vi "FlexibleBlock - Finite PCM Acquisition(Slave) - I2S.vi"() -> ()   [LabVIEW 2021]
uses:
  <vilib>/PDM Acquisition Toolkit/host/Classes/Session/Controls/Logic Levels.ctl
  <vilib>/PDM Acquisition Toolkit/shared/controls/PCM Data Format Configuration.ctl
  <vilib>/PDM Acquisition Toolkit/shared/controls/Digital Edge.ctl
  <vilib>/PDM Acquisition Toolkit/shared/controls/PCM Bit Endianness.ctl
  <vilib>/PDM Acquisition Toolkit/shared/controls/PCM Data Justification.ctl
  <vilib>/PDM Acquisition Toolkit/shared/controls/PCM Frame Sync Control.ctl
  Program Files/National Instruments/LabVIEW 2021/examples/PDM Acquisition Toolkit/subVIs/PCM Interface Type.ctl
  Users/Admin/Desktop/Release audio branch/Audio/audio_d/audio_MeasurementService/source/measurements/ac/audio_acMeasurement/Measurement Results.ctl
  <vilib>/addons/_NISVFA/_Shared subVIs/Controls/svc_Window.ctl
  <vilib>/PDM Acquisition Toolkit/host/Classes/Tasks/PDM Tasks/Controls/Acquisition Mode.ctl
  <vilib>/addons/_NISVFA/_Shared subVIs/Common/SVL Set dB Reference (N Ch - 1 Ref).vi
  <vilib>/addons/Sound and Vibration/svt_Level/SVL AC & DC Level (Time) (N Ch).vi
  <vilib>/addons/Sound and Vibration/svt_Single Tone Measurements/SVT Spurious Free Dynamic Range (Frequency) (1 Ch).vi
  <vilib>/addons/_NISVFA/_Spectrum Processing/SVFA Unit Conversion (Complex) (1 Ch).vi
  <vilib>/addons/_NISVFA/_Shared subVIs/Common/SVL Set dB Reference (1 Ch).vi
  <vilib>/addons/Sound and Vibration/svt_Level/SVL AC & DC Level (Time) (1 Ch).vi
  <vilib>/addons/_NISVFA/_Spectrum Processing/SVFA Get Spectrum Subset.vi
  <vilib>/addons/_NISVFA/_Spectrum Processing/SVFA Get Spectrum Subset (Complex) (1 Ch).vi
  <vilib>/addons/_NISVFA/_Shared subVIs/Common/svc_Window Parameters.vi
  <vilib>/addons/_NISVFA/_Shared subVIs/Common/svc_Extract Single Tone Information (complex).vi
  <vilib>/addons/_NISVFA/_Shared subVIs/Common/svc_Check Frequency Range in Spectrum.vi
  <vilib>/addons/_NISVFA/_Spectrum Processing/SVFA Spectrum Peak Search.vi
  <vilib>/addons/_NISVFA/_Spectrum Processing/SVFA Spectrum Peak Search (1 Ch).vi
  <vilib>/addons/_NISVFA/_Shared subVIs/Common/svc_Spectrum Units.vi
  <vilib>/addons/_NISVFA/_Shared subVIs/Common/svc_Log View for Spectrum (1Ch).vi
  <vilib>/addons/_NISVFA/_Spectrum Processing/SVFA Unit Conversion (1 Ch).vi
  <vilib>/addons/_NISVFA/_Shared subVIs/Common/svc_Complex Datatype Defaults.vi
  <vilib>/addons/_NISVFA/_Shared subVIs/Common/svc_Build Unit Label for Frequency Range.vi
  <vilib>/addons/_NISVFA/_Shared subVIs/Common/SVL Set dB Reference (variant).vi
  <vilib>/addons/_NISVFA/_Shared subVIs/Common/svc_Get SV Channel Info.vi
  <vilib>/Analysis/baseanly.llb/Mean.vi
  <vilib>/Analysis/baseanly.llb/Mean (DBL).vi
  <vilib>/addons/_NISVFA/_Shared subVIs/Windowing/svfa_Scaled Time Domain Window (Array).vi
  <vilib>/addons/_NISVFA/_Spectrum Processing/SVFA Get Tone Amplitude and Phase (1 Ch).vi
  <vilib>/addons/_NISVFA/_Spectrum Processing/subVIs/svfa_Compute Complex Spectrum for Export.vi
  <vilib>/addons/_NISVFA/_Shared subVIs/Common/svc_Check Frequency Range in Bandwidth.vi
  <vilib>/addons/_NISVFA/_Shared subVIs/Common/svc_Convert Start and Stop to Start Index and Length.vi
  <vilib>/addons/_NISVFA/_Spectrum Processing/subVIs/svfa_Spectrum Peak Search.vi
  <vilib>/addons/_NISVFA/_Shared subVIs/Common/svc_Format Value (DBL).vi
  <vilib>/addons/_NISVFA/_Shared subVIs/Common/svc_Get Weighting Enum and Labels.vi
  <vilib>/addons/_NISVFA/_Shared subVIs/Common/svc_Engineering Units to Unit Label.vi
  <vilib>/addons/_NISVFA/_Shared subVIs/Common/svc_Surround NonAlpha String with Parentheses.vi
  <vilib>/dlg_ctls.llb/Space Constant.vi
  <vilib>/addons/_NISVFA/_Shared subVIs/Common/svc_Unwrap Phase.vi
  <vilib>/addons/_NISVFA/_Shared subVIs/Common/svc_Convert Spectrum Array to dB.vi
  <vilib>/addons/_NISVFA/_Spectrum Processing/subVIs/svfa_Conversion Utility (spectrum info).vi
  <vilib>/addons/_NISVFA/_Shared subVIs/Common/svc_Unit Label to Engineering Units.vi
  <vilib>/addons/_NISVFA/_Spectrum Processing/subVIs/svfa_Spectrum Info Window to windowTd Type Def.vi
  <vilib>/Analysis/4window.llb/Force Window.vi
  <vilib>/Analysis/4window.llb/Force Window (DBL).vi
  <vilib>/Analysis/4window.llb/Exponential Window.vi
  <vilib>/Analysis/4window.llb/Exponential Window (DBL).vi
  <vilib>/addons/_NISVFA/_Spectrum Processing/subVIs/svfa_Window Frequency Response.vi
  <vilib>/addons/_NISVFA/_Spectrum Processing/subVIs/svfa_Window Frequency Response (double array).vi
  <vilib>/Analysis/baseanly.llb/Dot Product.vi
  <vilib>/Analysis/baseanly.llb/Complex Dot Product.vi
  <vilib>/addons/_NISVFA/_Spectrum Processing/subVIs/svfa_Peak Rough Search Indices.vi
  <vilib>/addons/_NISVFA/_Shared subVIs/Common/svc_Unit Label Lexical Class.vi
  <vilib>/addons/_NISVFA/_Spectrum Processing/subVIs/svfa_Peak to RMS to Peak2Peak.vi
  <vilib>/addons/_NISVFA/_Spectrum Processing/subVIs/svfa_Mag to Mag2.vi
  <vilib>/addons/_NISVFA/_Spectrum Processing/subVIs/svfa_Linear to dB.vi
  <vilib>/addons/_NISVFA/_Spectrum Processing/subVIs/svfa_dBrefA to dBrefB.vi
  <vilib>/addons/_NISVFA/_Spectrum Processing/subVIs/svfa_Spectrum to Spectral Density.vi
  <vilib>/addons/_NISVFA/_Spectrum Processing/subVIs/svfa_Rect Window Frequency Response.vi
  <vilib>/addons/_NISVFA/_Spectrum Processing/subVIs/svfa_Cosine Window Coefficients.vi
  <vilib>/PDM Acquisition Toolkit/host/API/Public/Create Tasks/Create PCM Input Task.vi
  <vilib>/PDM Acquisition Toolkit/host/API/Public/Configure/Timing/Configure Timing - PCM Input Slave.vi
  <vilib>/PDM Acquisition Toolkit/host/API/Public/Configure/PDM Channel/Configure Microphone Sensitivity FSPA - PCM Input Task.vi
  <vilib>/PDM Acquisition Toolkit/host/API/Public/Utility/Configure Simulation Mode - PCM Input Task.vi
  <vilib>/PDM Acquisition Toolkit/host/API/Public/Start/Start PCM Input Task.vi
  <vilib>/PDM Acquisition Toolkit/host/API/Public/Read/Read PCM Input Waveform.vi
  <vilib>/measure/matone.llb/Extract Single Tone Information N Chan.vi
  <vilib>/PDM Acquisition Toolkit/host/API/Public/Clear/Clear PCM Input Task.vi
  <vilib>/addons/Sound and Vibration/svt_Weighting/SVT Weighting Filter (N Ch).vi
  <vilib>/addons/_NISVFA/_Shared subVIs/Common/svc_Caller VI Returned in Error Source.vi
  <vilib>/addons/_NISVFA/_Shared subVIs/Common/svc_Get Window Info.vi
  <vilib>/Analysis/0measdsp.llb/Scaled Time Domain Window.vi
  <vilib>/Analysis/0measdsp.llb/Scaled Time Domain Window (DBL).vi
  <vilib>/Utility/error.llb/Error Cluster From Error Code.vi
  <vilib>/Analysis/baseanly.llb/Std Deviation and Variance.vi
  <vilib>/addons/Sound and Vibration/svt_Single Tone Measurements/SVT Gain (Time) (1 Ch).vi
  <vilib>/addons/Sound and Vibration/svt_Distortion/SVT SNR without Harmonics (Frequency) (1 Ch).vi
  <vilib>/addons/Sound and Vibration/svt_Single Tone Measurements/SVT Dynamic Range (Frequency) (1 Ch).vi
  <vilib>/addons/Sound and Vibration/svt_Distortion/subVIs/sv_Check Data Valid (Audio) (1 Ch).vi
  <vilib>/addons/_NISVFA/_Shared subVIs/Common/svc_Convert Frequency to Frequency String.vi
  <vilib>/Analysis/4window.llb/window parameters.vi
  <vilib>/Analysis/4window.llb/Window Properties.vi
  <vilib>/Analysis/4window.llb/Window Properties by Name.vi
  <vilib>/addons/_NISVFA/_Spectrum Processing/subVIs/svfa_Spectrum Peak Tone Search and Estimation (complex).vi
  <vilib>/measure/masignal.llb/Tones and Noise Waveform.vi
  <vilib>/addons/_NISVFA/_Shared subVIs/Common/svc_FFT with Window.vi
  <vilib>/Analysis/1siggen.llb/Square Wave.vi
  <vilib>/addons/_NISVFA/_Spectrum Processing/subVIs/svfa_Three Finger Peak Search.vi
  <vilib>/addons/Sound and Vibration/svt_Distortion/subVIs/sv_Peak View Amplitude (1 Ch).vi
  <vilib>/PDM Acquisition Toolkit/host/API/PDM Acquisition Toolkit.lvlib
  <vilib>/PDM Acquisition Toolkit/host/Classes/Tasks/PDM Tasks/PDM Task.lvclass
  <vilib>/measure/NI_MAPro.lvlib
  <vilib>/addons/Sound and Vibration/svt_Single Tone Measurements/SoundVib_SingleTone.lvlib
  <vilib>/addons/Sound and Vibration/svt_Distortion/SoundVib_Distortion.lvlib
  <vilib>/addons/Sound and Vibration/svt_Weighting/SoundVib_ABCWeighting.lvlib
  <vilib>/PDM Acquisition Toolkit/host/Classes/Session/DecoderSession.lvclass
  <vilib>/PDM Acquisition Toolkit/shared/PDM Shared.lvlib
  Users/Admin/Desktop/Release audio branch/Audio/audio_d/audio_MeasurementService/source/measurements/ac/audio_acMeasurement/audio_acMeasurement.lvlib
panel:
  out "FreqDomainGraph":cluster{"x0":dbl, "dx":dbl, "magnitude":dbl[]}(graph) caption="AC"
  out "output cluster":T1
  out "error out":errorcluster
  in  "Latch Delay(ns)":sgl
  in  "PCM Interfaces":T2
  out "elements remaining":u32[](array[numeric])=[26]
  out "Frame Sync Clock Control":T3={"Frame Length"=64, "Frame Sync Pulse Width"=32, "Bit Clock Edge  Sync"=enum."Falling"}
  out "PCM Data Configuration":T5={"Frame Sync Edge for Channel 0"=enum."Falling", "Channel Count Per Frame"=2, "Channel Length"=32, "Bit Depth"=24, "Channel 0 Offset"=1, "Endianness"=enum."MSB First", "Data Justification"=enum."Left Justified"}
  in  "Bit clock rate":u32=12288000 format="%.4p"
  in  "logic level":T8
  out "Requested Sampling Rate":dbl=192000.0 format="%#_6p"
  out "detected phases (deg)":dbl[](array[numeric])=[48.77177137902379, 163.50683535190996] format="%.2p"
  out "detected amplitudes":dbl[](array[numeric])=[0.002127835538874218, 39.382575869286214] format="%.2p"
  out "detected frequencies":dbl[](array[numeric])=[87725.90443160792, 99.99819936214169] format="%.2p"
  in  "simulation mode":bool
  out "PCM Data":waveform(dbl)[](graph)=[{"t0"=timestamp(0 s since 1904-01-01), "dt"=5.208333277550992e-06, "Y"=array[4000 elements], "attributes"=variant("NI_ChannelName"=variant(string "PCMI0.0"))}, {"t0"=timestamp(0 s since 1904-01-01), "dt"=5.208333277550992e-06, "Y"=array[4000 elements], "attributes"=variant("NI_ChannelName"=variant(string "PCMI0.1"))}]
  in  "microphone sensitivity (dB/Pa)":dbl=0.34762
  in  "number of words":i32=19200
  in  "channel list":string="7820\\PCMi 0"
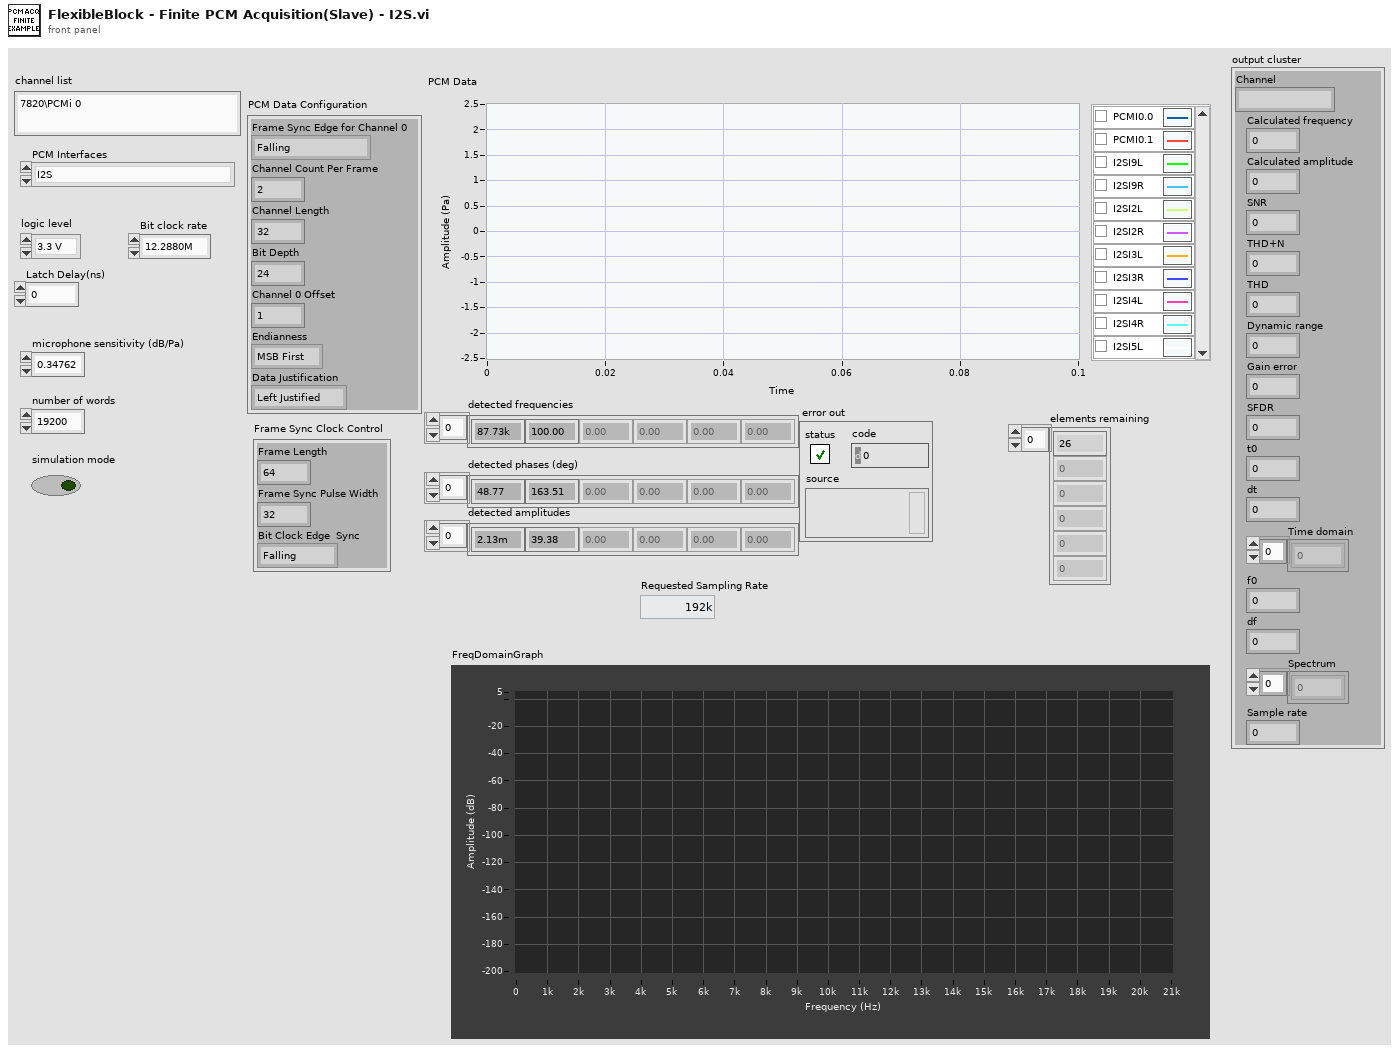
[diagram p1: front panel]
types:
  T1 = typedef "audio_acMeasurement.lvlib/Measurement Results.ctl" = cluster{"Channel":string, "Calculated frequency":dbl, "Calculated amplitude":dbl, "SNR":dbl, "THD+N":dbl, "THD":dbl, "Dynamic range":dbl, "Gain error":dbl, "SFDR":dbl, "t0":dbl, "dt":dbl, "Time domain":dbl[], "f0":dbl, "df":dbl, "Spectrum":dbl[], "Sample rate":u32}
  T2 = typedef "PCM Interface Type.ctl" = enum16{"I2S", "Left Justified", "Right Justified", "TDM 4 Channel", "TDM 6 Channel", "TDM 8 Channel", "DSP mode", "DSP mode with 1 bit delay", "PCM Short Frame", "PCM Long Frame"}
  T3 = typedef "PDM Shared.lvlib/PCM Frame Sync Control.ctl" = cluster{"Frame Length":u16, "Frame Sync Pulse Width":u16, "Bit Clock Edge  Sync":T4}
  T4 = typedef "PDM Shared.lvlib/Digital Edge.ctl" = enum8{"Rising", "Falling"}
  T5 = typedef "PDM Shared.lvlib/PCM Data Format Configuration.ctl" = cluster{"Frame Sync Edge for Channel 0":T4, "Channel Count Per Frame":u8, "Channel Length":u16, "Bit Depth":u8, "Channel 0 Offset":u16, "Endianness":T6, "Data Justification":T7}
  T6 = typedef "PDM Shared.lvlib/PCM Bit Endianness.ctl" = enum16{"MSB First", "LSB First"}
  T7 = typedef "PDM Shared.lvlib/PCM Data Justification.ctl" = enum16{"Left Justified", "Right Justified"}
  T8 = typedef "PDM Acquisition Class Library.lvlib/DecoderSession.lvclass/Logic Levels.ctl" = enum16{"3.3 V", "1.8 V", "1.2 V"}
  T9 = cluster{"Channel":string, "Calculated frequency":dbl, "Calculated amplitude":dbl, "SNR":dbl, "THD+N":dbl, "THD":dbl, "Dynamic range":dbl, "Gain error":dbl, "SFDR":dbl, "t0":dbl, "dt":dbl, "Time domain":dbl[], "f0":dbl, "df":dbl, "Spectrum":dbl[], "Sample rate":u32}
  T10 = enum16{"no change", "spectrum", "spectral density"}
  T11 = cluster{"linear/dB":enum16{"no change", "linear", "dB"}, "dB reference (0: no change)":dbl, "power/magnitude":enum16{"no change", "power", "magnitude"}, "view":enum16{"no change", "rms", "peak", "peak-peak"}}
  T12 = cluster{"start frequency":dbl, "stop frequency":dbl}
  T13 = cluster{"gain units":enum16{"dB", "linear ratio"}, "detected fundamental amplitude units":enum16{"EU rms", "EU peak", "EU peak-peak"}}
  T14 = typedef "svc_Window.ctl" = u32
  T15 = cluster{"SNR units":enum16{"dB", "linear ratio", "%"}, "detected fundamental amplitude units":enum16{"EU rms", "EU peak", "EU peak-peak"}}
  T16 = typedef "PDM Acquisition Class Library.lvlib/PDM Task.lvclass/Acquisition Mode.ctl" = enum16{"Finite", "Continuous"}
  T17 = typedef "PDM Acquisition Class Library.lvlib/PCM Input Task.lvclass/DVR PCM Input Task.ctl" = refnum<data-value>
  T18 = typedef "svc_Spectrum Info.ctl" = cluster{"channel name":string, "description":string, "x-axis units":T19, "spectral info":cluster{"spectrum type":T20, "linear/dB":enum16{"linear", "dB"}, "window":u16, "window size":i32, "FFT size":i32}, "engineering units":T21, "custom label":string, "dB reference [EU]":dbl, "peak units":enum16{"rms", "peak", "peak-peak"}, "weighting filter":T22, "spectral density?":bool, "unit label":string, "spectrum skewed?":bool, "complimentary spectrum units":T23}
  T19 = typedef "svc_X-Axis Units.ctl" = u16
  T20 = typedef "svc_Spectrum Type.ctl" = enum16{"FFT Spectrum [complex]", "Amplitude [Magnitude]", "Power [Magnitude^2]", "Cross Spectrum [complex]", "Frequency Response [Complex]"}
  T21 = typedef "svc_Engineering Units Text Ring.ctl" = u16
  T22 = typedef "svc_Weighting Filter Text Ring.ctl" = u16
  T23 = typedef "svc_Complimentary Spectrum Units.ctl" = enum16{"none", "radians", "degrees", "cycles", "imaginary"}
  T24 = cluster{"complex spectrum response":cluster{"f0":dbl, "df":dbl, "complex spectrum":cdb[]}, "spectrum info":T18}
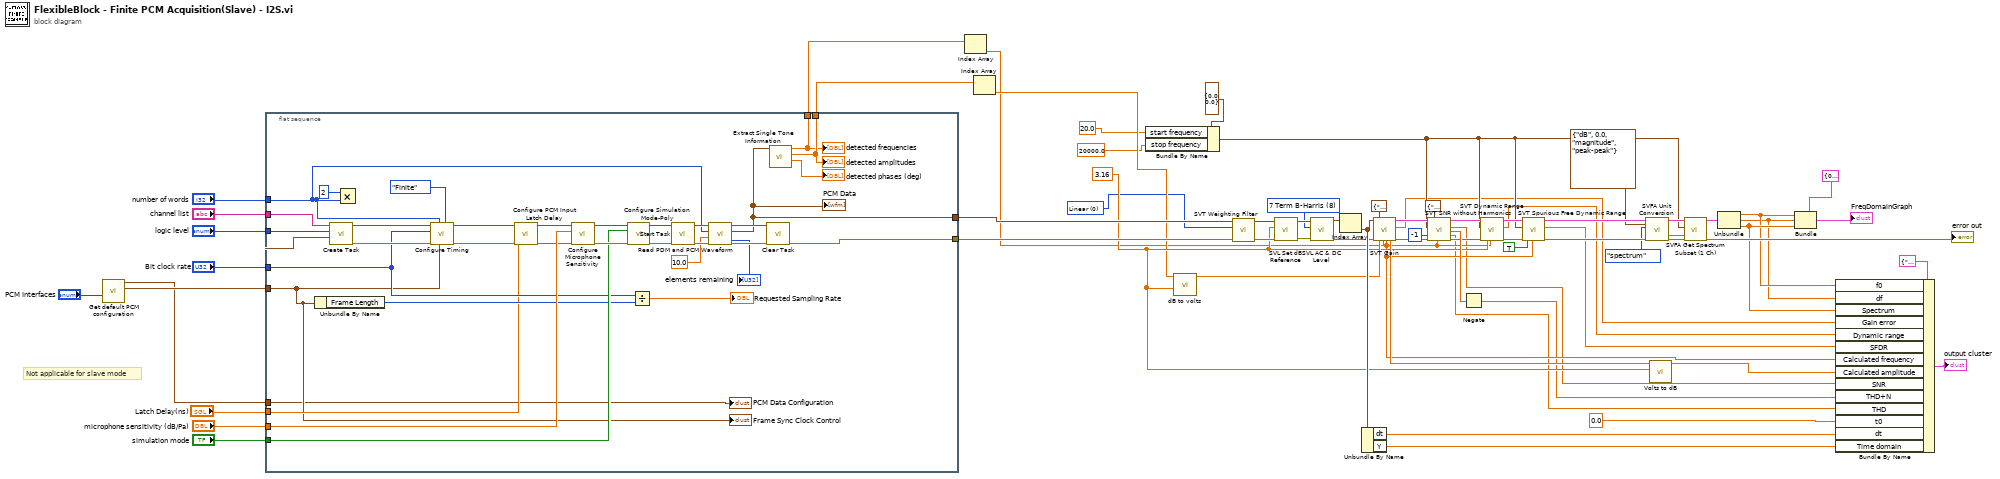
[diagram p0: block diagram]
diagram:
  w21 = u16 0 items=["Linear", "A-weighting", "B-weighting", "C-weighting"] ("weighting")
  w24 = 3.16 ("start frequency")
  w44 = T14 8 items=["None"=0, "Hanning"=1, "Hamming"=2, "Blackman-Harris"=3, "Exact Blackman"=4, "Blackman"=5, "Flat Top"=6, "4 Term B-Harris "=7, "7 Term B-Harris"=8, "Low Sidelobe"=9, "Force"=64, "Exponential"=65, "Blackman Nuttall"=11, "Triangle"=30, "Bartlett-Hanning"=31, "Bohman"=32, "Parzen"=33, "Welch"=34, "Kaiser"=60, "Dolph-Chebyshev"=61, "Gaussian"=62] ("window")
  # "Not applicable for slave mode"
  n1 = call "Get default PCM configuration.vi"("PCM Interfaces"="PCM Interfaces") -> ("Frame Sync Clock Control"=w62:T3, "PCM Data Configuration"=w61:T5)  [unwired: 9 in]
  n2 = flat-sequence {
    tunnel: "logic level" -> [w104]
    tunnel: "channel list" -> [w103]
    tunnel: "microphone sensitivity (dB/Pa)" -> [w101]
    tunnel: "simulation mode" -> [w94]
    tunnel: "Bit clock rate" -> [w85]
    tunnel: "number of words" -> [w78]
    tunnel: "Latch Delay(ns)" -> [w77]
    tunnel: w62 -> [w76]
    tunnel: w61 -> [w75]
    tunnel: [w74] -> w28
    tunnel: [w73] -> w27
    tunnel: [w72] -> w26
    tunnel: [w71] -> w25
    frame #0 {
      n3 = Unbundle By Name(w76) -> ("Frame Length"=w81:u16)
      n4 = call-poly <vilib>:"Create Task.vi"("PCM data configuration"=w75, "logic level"=w104, "channel list"=w103) -> ("error out"=w92:errorcluster, "PCM input task out"=w91:T17)  [unwired: 7 in]
      n5 = Multiply(x=2, y=w78) -> ()  [unwired: 1 out]
      n6 = call-poly <vilib>:"Configure Timing.vi"("acquisition mode"=Acquisition_Mode."Finite", "Frame Sync Clock Control"=w76, "number of words per channel"=w78, "error in"=w92, "Bit Clock rate"=w85, "PCM input task in"=w91) -> ("error out"=w90:errorcluster, "PCM input task out"=w83:T17)  [unwired: 4 in]
      n7 = call <vilib>:"Configure PCM Input Latch Delay.vi"("error in"=w90, "Latch Delay(ns)"=w77, "PCM input task in"=w83) -> ("error out"=w89:errorcluster, "PCM input task out"=w88:T17)  [unwired: 6 in, 1 out]
      n8 = call-poly <vilib>:"Configure Microphone Sensitivity.vi"("error in"=w89, "microphone sensitivity (FS/Pa)"=w101, "PCM input task in"=w88) -> ("error out"=w96:errorcluster, "PCM input task out"=w95:T17)  [unwired: 7 in]
      n9 = call-poly <vilib>:"Configure Simulation Mode-Poly.vi"("error in"=w96, "simulation mode"=w94, "PCM Input Task in"=w95) -> ("error out"=w86:errorcluster, "PCM Input Task out"=w87:T17)  [unwired: 7 in]
      n10 = Divide(x=w85, y=w81) -> (x/y=→"Requested Sampling Rate":dbl)
      n11 = call-poly <vilib>:"Start Task.vi"("error in"=w86, "PCM input task in"=w87) -> ("error out"=w100:errorcluster, "PCM input task out"=w99:T17)  [unwired: 8 in]
      n12 = call-poly <vilib>:"Read PDM and PCM Waveform.vi"("error in"=w100, "timeout"=10.0, "words per channel"=w78, "PCM input task In"=w99) -> ("error out"=w98:errorcluster, "PCM waveforms"=w73:waveform(dbl)[], "PCM input task out"=w97:T17, "elements remaining"=→"elements remaining":u32[])  [unwired: 4 in]
      "PCM Data" <- w73
      n13 = call-poly <vilib>:"Clear Task.vi"("error in"=w98, "PCM input task in"=w97) -> ("error out"=w74:errorcluster)  [unwired: 9 in]
      n14 = call-poly <vilib>:"Extract Single Tone Information.vi"("time signals in"=w73) -> ("detected phases (deg)"=→"detected phases (deg)":dbl[], "detected amplitudes"=w72:dbl[], "detected frequencies"=w71:dbl[])  [unwired: 5 in, 3 out]
      "detected frequencies" <- w71
      "detected amplitudes" <- w72
      "PCM Data Configuration" <- w75
      "Frame Sync Clock Control" <- w76
    }
  }
  n15 = Index Array(array=w25) -> (element=w22:dbl)  [unwired: 1 in]
  n16 = Index Array(array=w26) -> (element=w23:dbl)  [unwired: 1 in]
  n17 = Bundle By Name(cluster=T12 {"start frequency"=0.0, "stop frequency"=0.0} ("frequency range"), "start frequency"=20.0, "stop frequency"=20000.0 ("start frequency")) -> (w33:T12)
  n18 = call "dB to volts.vi"("Full scale range"=w24, "Voltage(dB)"=w23) -> ("Voltage(volts)"=w37:dbl)  [unwired: 9 in]
  n19 = call-poly <vilib>:"SVT Weighting Filter.vi"("error in (no error)"=w28, "weighting"=w21, "scaled signals [EU]"=w27) -> ("error out"=w58:errorcluster, "weighted signals [EU]"=w57:waveform(dbl)[])  [unwired: 6 in]
  n20 = call-poly <vilib>:"SVL Set dB Reference.vi"("error in (no error)"=w58, "dB reference [EU]"=w24, "scaled signals in [EU]"=w57) -> ("error out"=w45:errorcluster, "scaled signals out [EU]"=w47:waveform(dbl)[])  [unwired: 7 in]
  n21 = call-poly <vilib>:"SVL AC & DC Level.vi"("scaled signals in [EU]"=w47, "window"=w44, "error in (no error)"=w45) -> ("AC signals [EU]"=w46:waveform(dbl)[], "error out"=w53:errorcluster)  [unwired: 11 in, 4 out]
  n22 = Index Array(array=w46) -> (element=w60:waveform(dbl))  [unwired: 1 in]
  n23 = Unbundle By Name(w60) -> ("dt"=w15:dbl, "Y"=w14:dbl[])
  n24 = call-poly <vilib>:"SVT Gain.vi"("scaled signal [EU]"=w60, "error in (no error)"=w53, "desired units"=T13 {"gain units"=enum."dB", "detected fundamental amplitude units"=enum."EU peak"}, "amplitude [EU peak]"=w37, "expected fundamental frequency [Hz]"=w22) -> ("detected fundamental\nfrequency [Hz]"=w20:dbl, "detected fundamental\namplitude"=w36:dbl, "complex spectrum"=w42:T24, "gain"=w4:dbl, "error out"=w43:errorcluster)  [unwired: 9 in, 1 out]
  n25 = call-poly <vilib>:"SVT SNR without Harmonics.vi"("complex spectrum"=w42, "frequency range"=w33, "maximum harmonic"=-1, "error in (no error)"=w43, "desired units"=T15 {"SNR units"=enum."dB", "detected fundamental amplitude units"=enum."EU rms"}, "expected fundamental frequency [Hz]"=w20) -> ("complex spectrum"=w49:T24, "SNR (without harmonics)"=w19:dbl, "SINAD"=w50:dbl, "THD"=w17:dbl, "error out"=w48:errorcluster)  [unwired: 6 in, 3 out]
  n26 = Negate(x=w50) -> (-x=w18:dbl)
  n27 = call-poly <vilib>:"SVT Dynamic Range.vi"("complex spectrum"=w49, "frequency range"=w33, "error in (no error)"=w48, "full scale amplitude [EU peak]"=w24, "expected fundamental\nfrequency [Hz]"=w20) -> ("dup complex spectrum"=w54:T24, "dynamic range"=w1:dbl, "error out"=w55:errorcluster)  [unwired: 9 in, 3 out]
  n28 = call-poly <vilib>:"SVT Spurious Free Dynamic Range.vi"("complex spectrum"=w54, "frequency range"=w33, "error in (no error)"=w55, "exclude harmonics"=TRUE, "expected fundamental\nfrequency [Hz]"=w20) -> ("complex spectrum"=w40:T24, "spurious free dynamic range"=w2:dbl, "error out"=w41:errorcluster)  [unwired: 7 in, 5 out]
  n29 = call-poly <vilib>:"SVFA Unit Conversion.vi"("complex spectrum"=w40, "desired scaling"=T11 {"linear/dB"=enum."dB", "dB reference (0: no change)"=0.0, "power/magnitude"=enum."magnitude", "view"=enum."peak-peak"}, "spectral density desired"=T10."spectrum", "error in (no error)"=w41) -> ("converted spectrum"=w34:cluster{"x0":dbl, "dx":dbl, "magnitude":dbl[]}, "spectrum info out"=w30:T18, "error out"=w29:errorcluster)  [unwired: 10 in, 3 out]
  n30 = call "Volts to dB.vi"("Full scale range"=w24, "Voltage(V)"=w36) -> ("Voltage(dB)"=w3:dbl)  [unwired: 9 in]
  n31 = call <vilib>:"SVFA Get Spectrum Subset (1 Ch).vi"("spectrum"=w34, "range"=w33, "spectrum info"=w30, "error in (no error)"=w29) -> ("spectrum subset"=w32:cluster{"x0":dbl, "dx":dbl, "magnitude":dbl[]}, "error out"=→"error out":errorcluster)  [unwired: 10 in, 4 out]
  n32 = Unbundle(w32) -> ("x0"=w8:dbl, "dx"=w5:dbl, "magnitude"=w9:dbl[])
  n33 = Bundle(cluster=cluster{"x0":dbl, "dx":dbl, "magnitude":dbl[]} {"x0"=0.0, "dx"=0.0, "magnitude"=[]} ("FreqDomainGraph"), "x0"=w8, "dx"=w5, "magnitude"=w9) -> (→"FreqDomainGraph":cluster{"x0":dbl, "dx":dbl, "magnitude":dbl[]})
  n34 = Bundle By Name(cluster=T9 {"Channel"="", "Calculated frequency"=0.0, "Calculated amplitude"=0.0, "SNR"=0.0, "THD+N"=0.0, "THD"=0.0, "Dynamic range"=0.0, "Gain error"=0.0, "SFDR"=0.0, "t0"=0.0, "dt"=0.0, "Time domain"=[], "f0"=0.0, "df"=0.0, "Spectrum"=[], "Sample rate"=0} ("Measurement Results"), "f0"=w8, "df"=w5, "Spectrum"=w9, "Gain error"=w4, "Dynamic range"=w1, "SFDR"=w2, "Calculated frequency"=w20, "Calculated amplitude"=w3, "SNR"=w19, "THD+N"=w18, "THD"=w17, "t0"=0.0 ("Wfm t0"), "dt"=w15, "Time domain"=w14) -> (→"output cluster":T9)
